vi "Start Game.vi"(8 "error in (no error)":errorcluster) -> (0 "error out":errorcluster, 2 "Board Size out":i16)   [LabVIEW 2017]
panel:
  in  "OK":bool
  in  "Board Size":i16=4
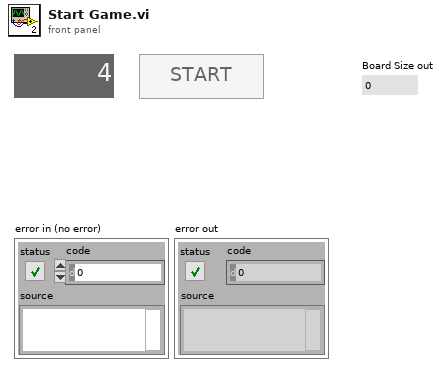
[diagram p1: front panel]
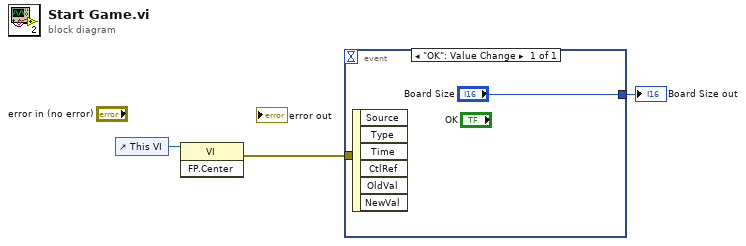
[diagram p0: block diagram]
diagram:
  n1 = control-ref of="This VI"() -> (w3:refnum<vi>)
  n2 = invoke class="VI" method="FP.Center"(reference=w3) -> (error out=w2:errorcluster)  [unwired: 2 in, 2 out]
  n3 = event shown="[0] \"OK\": Value Change" {
    selector: _ -> [_]
    dyn-events: _ -> [_]
    timeout: _ -> [_]
    tunnel: w2 -> [_]
    tunnel: ["Board Size"] -> w1
    event "OK": Value Change {
      n4 = event-data() -> ()  [unwired: 1 in, 6 out]
    }
  }
  "Board Size out" <- w1
